vi "UI - All UI Objects Refs Memory.vi"(7 "Operation":T1, 8 "error in":errorcluster, 11 "VI Name (\"\" = Caller)":string) -> (0 "error out":errorcluster, 3 "Variant Out":variant)   [LabVIEW 2012]
uses:
  Controls/UI - All UI Objects Refs Memory - Operation.ctl
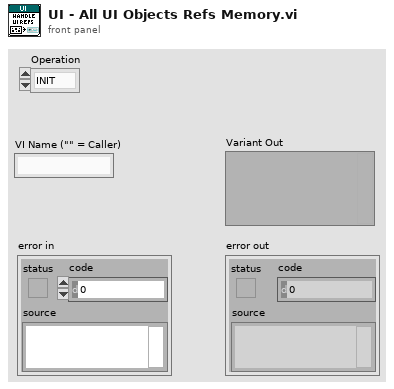
[diagram p1: front panel]
types:
  T1 = typedef "UI - All UI Objects Refs Memory - Operation.ctl" = enum16{"INIT", "GET", "ADD"}
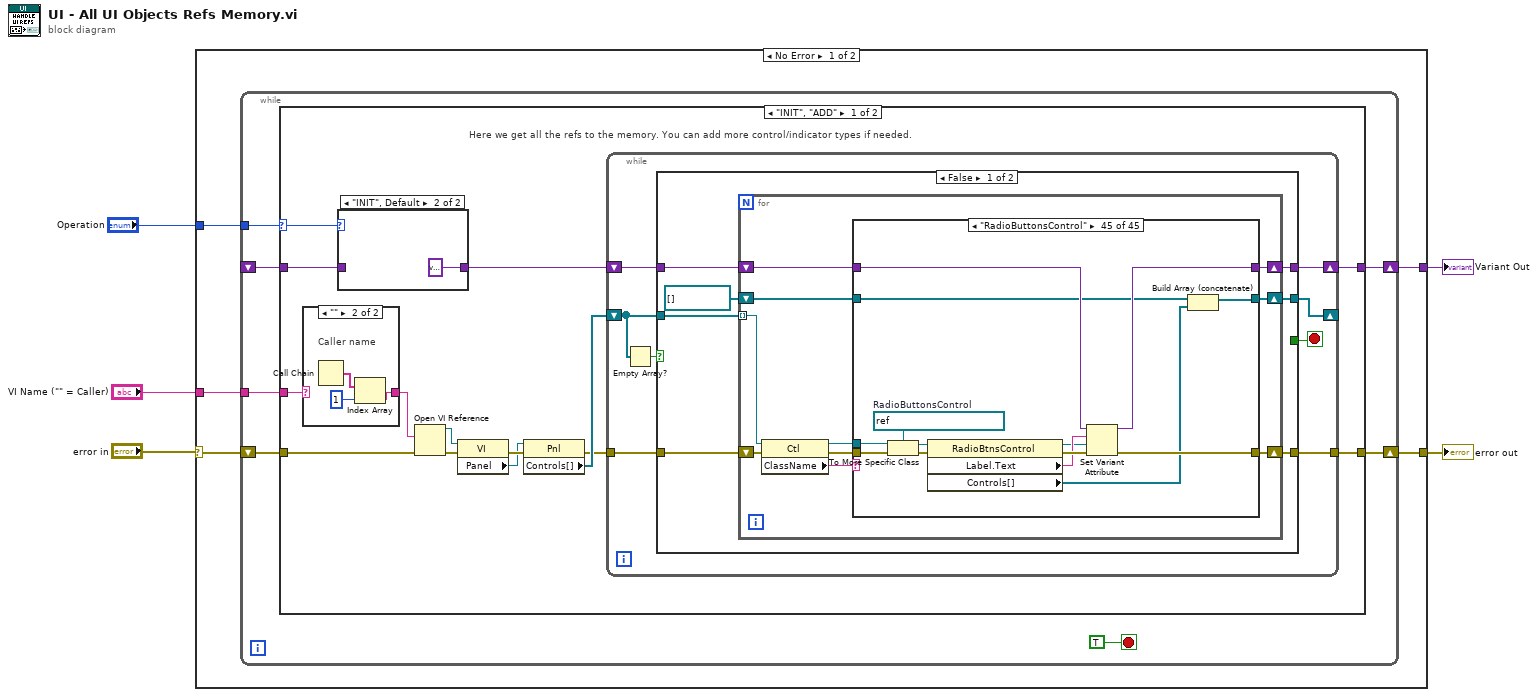
[diagram p0: block diagram]
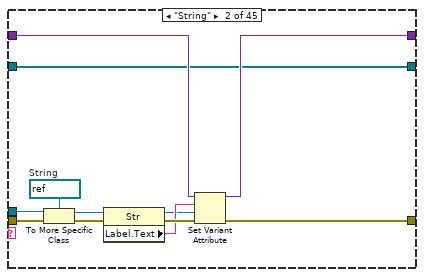
[diagram p3: hidden frame]
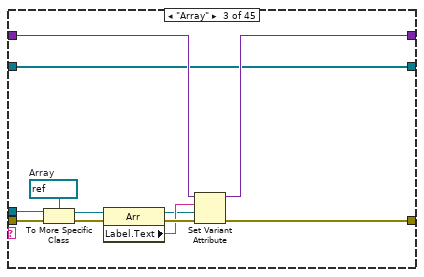
[diagram p4: hidden frame]
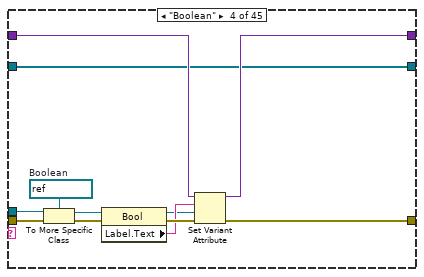
[diagram p5: hidden frame]
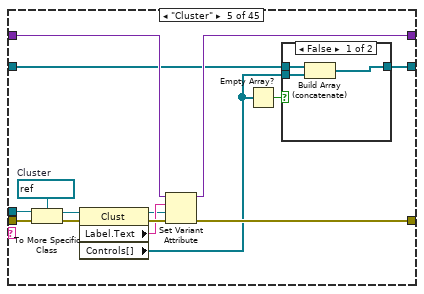
[diagram p6: hidden frame]
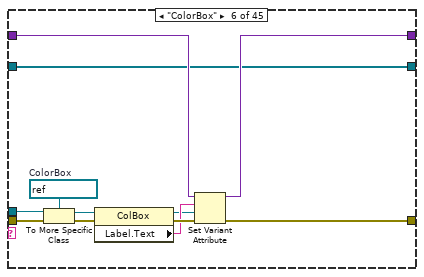
[diagram p8: hidden frame]
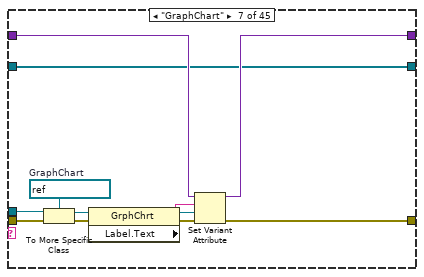
[diagram p9: hidden frame]
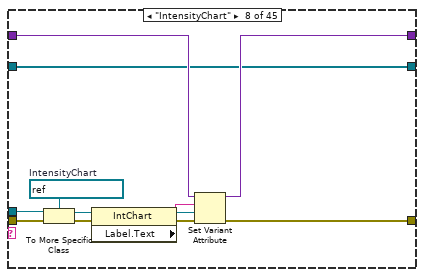
[diagram p10: hidden frame]
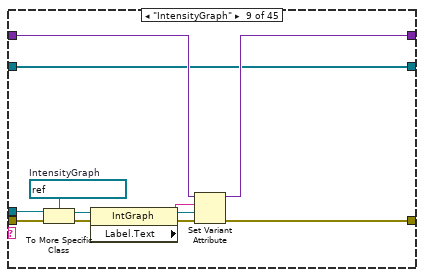
[diagram p11: hidden frame]
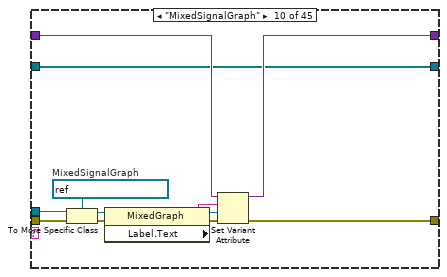
[diagram p12: hidden frame]
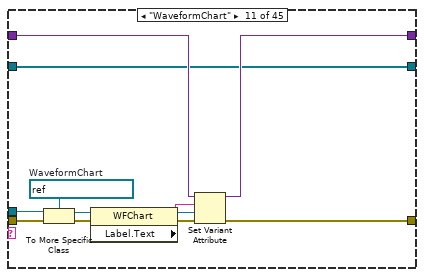
[diagram p13: hidden frame]
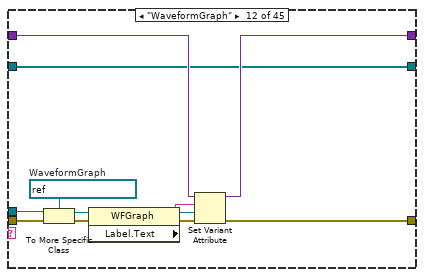
[diagram p14: hidden frame]
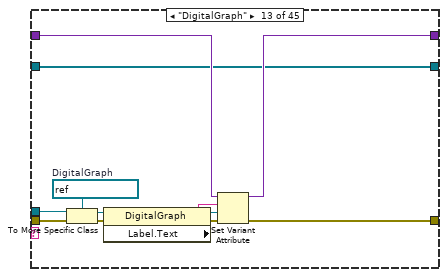
[diagram p15: hidden frame]
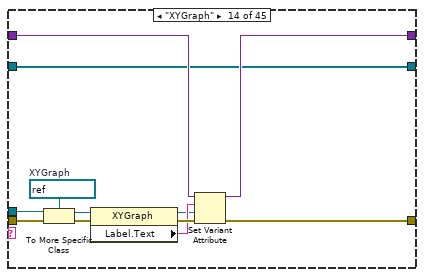
[diagram p16: hidden frame]
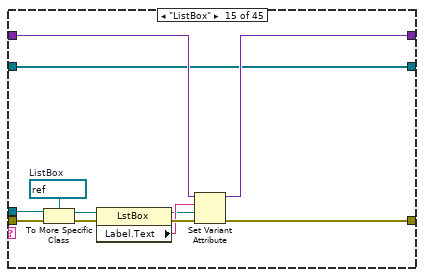
[diagram p17: hidden frame]
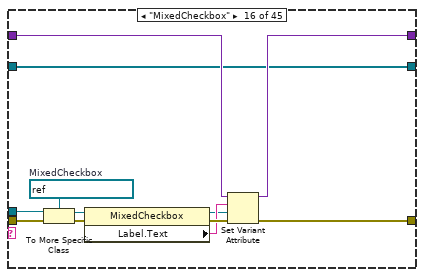
[diagram p18: hidden frame]
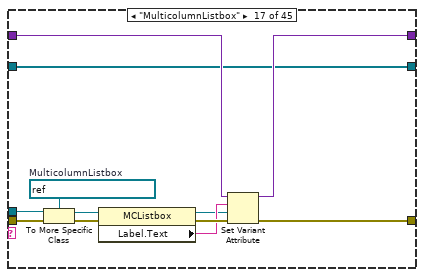
[diagram p19: hidden frame]
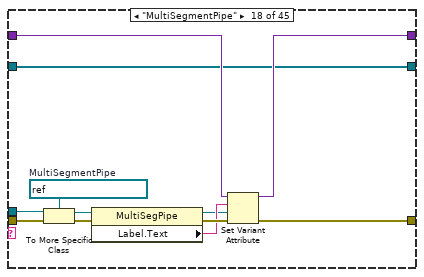
[diagram p20: hidden frame]
diagram:
  n1 = case shown="No Error" "error in" {
    selector: "error in" -> [w9 w617]
    tunnel: [w8 w617] -> w5
    tunnel: "Operation" -> [w10 _]
    tunnel: "VI Name (\"\" = Caller)" -> [w7 _]
    tunnel: [w6 _] -> w1
    frame No Error {
      n2 = while {
        tunnel: w10 -> [w16]
        shift-right: [w11] -> w8
        shift-left: w9 -> [w15]
        tunnel: w7 -> [w14]
        shift-right: [w13] -> w6
        shift-left: _ -> [w12]
        stop <- TRUE stop-if-true
        n3 = case shown="\"INIT\", \"ADD\"" w16 {
          selector: w16 -> [w20 _]
          tunnel: w15 -> [w31 w616]
          tunnel: w14 -> [w30 _]
          tunnel: [w22 w615] -> w13
          tunnel: w12 -> [w18 w615]
          tunnel: [w21 w616] -> w11
          frame "INIT", "ADD" {
            # "Here we get all the refs to the memory. You can add more control/indicator types if needed."
            n4 = case shown="\"\"" w30 {
              selector: w30 -> [w611 _]
              tunnel: [w611 w612] -> w29
              frame Default {
              }
              frame "" {
                # "Caller name"
                n5 = Call Chain() -> (call chain=w614:string[])
                n6 = Index Array(array=w614, index=1) -> (element=w612:string)
              }
            }
            n7 = case shown="\"INIT\", Default" w20 {
              tunnel: [w609 variant] -> w19
              tunnel: w18 -> [w609 _]
              frame "ADD" {
              }
              frame "INIT", Default {
              }
            }
            n8 = Open VI Reference(vi path=w29, error in (no error)=w31) -> (vi reference=w27:refnum<vi>, error out=w28:errorcluster)  [unwired: 4 in]
            n9 = property class="VI"(reference=w27, error in=w28) -> (error out=w26:errorcluster, "Panel"=w25:refnum<vi>)  [unwired: 1 out]
            n10 = property class="Pnl"(reference=w25, error in=w26) -> (error out=w23:errorcluster, "Controls[]"=w24:refnum<vi>[])  [unwired: 1 out]
            n11 = while {
              tunnel: w23 -> [w39]
              tunnel: [w37] -> w21
              shift-right: [w35] -> _
              shift-left: w24 -> [w34]
              shift-right: [w38] -> w22
              shift-left: w19 -> [w36]
              stop <- w32 stop-if-true
              n12 = Empty Array?(array=w34) -> (empty?=w33:bool)
              n13 = case shown="False" w33 {
                tunnel: w34 -> [w46 _]
                tunnel: w39 -> [w45 w608]
                tunnel: [w44 w607] -> w38
                tunnel: [w43 w608] -> w37
                tunnel: w36 -> [w42 w607]
                tunnel: [w41 _] -> w35
                tunnel: [_ TRUE] -> w32
                frame False {
                  n14 = for {
                    tunnel: w46 -> [w55] mode=indexing
                    shift-right: [w49] -> w43
                    shift-left: w45 -> [w56]
                    shift-right: [w51] -> w44
                    shift-left: w42 -> [w50]
                    shift-right: [w48] -> w41
                    shift-left: refnum<vi>[] [] ("Controls[]") -> [w47]
                    n15 = property class="Ctl"(reference=w55, error in=w56) -> (reference out=w52:refnum<vi>, error out=w54:errorcluster, "ClassName"=w53:string)
                    n16 = case shown="\"RadioButtonsControl\"" w53 {
                      tunnel: w54 -> [w58 w71 w83 w95 w110 w126 w138 w150 w162 w174 w186 w198 w210 w222 w234 w246 w258 w270 w282 w294 w306 w318 w330 w342 w354 w366 w378 w390 w405 w423 w435 w447 w459 w471 w483 w495 w507 w519 w531 w543 w555 w567 w579 w591 w605]
                      tunnel: w52 -> [_ w70 w82 w94 w109 w125 w137 w149 w161 w173 w185 w197 w209 w221 w233 w245 w257 w269 w281 w293 w305 w317 w329 w341 w353 w365 w377 w389 w404 w422 w434 w446 w458 w470 w482 w494 w506 w518 w530 w542 w554 w566 w578 w590 w604]
                      tunnel: [w59 w65 w77 w89 w104 w120 w132 w144 w156 w168 w180 w192 w204 w216 w228 w240 w252 w264 w276 w288 w300 w312 w324 w336 w348 w360 w372 w384 w399 w417 w429 w441 w453 w465 w477 w489 w501 w513 w525 w537 w549 w561 w573 w585 w599] -> w51
                      tunnel: w50 -> [w59 w64 w76 w88 w103 w119 w131 w143 w155 w167 w179 w191 w203 w215 w227 w239 w251 w263 w275 w287 w299 w311 w323 w335 w347 w359 w371 w383 w398 w416 w428 w440 w452 w464 w476 w488 w500 w512 w524 w536 w548 w560 w572 w584 w598]
                      tunnel: [w58 w61 w73 w85 w100 w116 w128 w140 w152 w164 w176 w188 w200 w212 w224 w236 w248 w260 w272 w284 w296 w308 w320 w332 w344 w356 w368 w380 w393 w413 w425 w437 w449 w461 w473 w485 w497 w509 w521 w533 w545 w557 w569 w581 w595] -> w49
                      tunnel: [w57 w60 w72 w84 w99 w115 w127 w139 w151 w163 w175 w187 w199 w211 w223 w235 w247 w259 w271 w283 w295 w307 w319 w331 w343 w355 w367 w379 w391 w412 w424 w436 w448 w460 w472 w484 w496 w508 w520 w532 w544 w556 w568 w580 w592] -> w48
                      tunnel: w47 -> [w57 w60 w72 w84 w98 w115 w127 w139 w151 w163 w175 w187 w199 w211 w223 w235 w247 w259 w271 w283 w295 w307 w319 w331 w343 w355 w367 w379 w392 w412 w424 w436 w448 w460 w472 w484 w496 w508 w520 w532 w544 w556 w568 w580 w593]
                      frame Default {
                        # "Not implemented"
                      }
                      frame "String" {
                        w67 = refnum<vi> refnum  # String
                        n17 = To More Specific Class(target class=w67, reference=w70, error in=w71) -> (specific class reference=w69:refnum<vi>, error out=w68:errorcluster)
                        n18 = property class="Str"(reference=w69, error in=w68) -> (reference out=w62:refnum<vi>, error out=w66:errorcluster, "Label.Text"=w63:string)
                        n19 = Set Variant Attribute(Variant=w64, name=w63, value=w62, error in=w66) -> (Variant out=w65:variant, error out=w61:errorcluster)  [unwired: 1 out]
                      }
                      frame "Array" {
                        w79 = refnum<vi> refnum  # Array
                        n20 = To More Specific Class(target class=w79, reference=w82, error in=w83) -> (specific class reference=w81:refnum<vi>, error out=w80:errorcluster)
                        n21 = property class="Arr"(reference=w81, error in=w80) -> (reference out=w74:refnum<vi>, error out=w78:errorcluster, "Label.Text"=w75:string)
                        n22 = Set Variant Attribute(Variant=w76, name=w75, value=w74, error in=w78) -> (Variant out=w77:variant, error out=w73:errorcluster)  [unwired: 1 out]
                      }
                      frame "Boolean" {
                        w91 = refnum<vi> refnum  # Boolean
                        n23 = To More Specific Class(target class=w91, reference=w94, error in=w95) -> (specific class reference=w93:refnum<vi>, error out=w92:errorcluster)
                        n24 = property class="Bool"(reference=w93, error in=w92) -> (reference out=w86:refnum<vi>, error out=w90:errorcluster, "Label.Text"=w87:string)
                        n25 = Set Variant Attribute(Variant=w88, name=w87, value=w86, error in=w90) -> (Variant out=w89:variant, error out=w85:errorcluster)  [unwired: 1 out]
                      }
                      frame "Cluster" {
                        w106 = refnum<vi> refnum  # Cluster
                        n26 = To More Specific Class(target class=w106, reference=w109, error in=w110) -> (specific class reference=w108:refnum<vi>, error out=w107:errorcluster)
                        n27 = property class="Clust"(reference=w108, error in=w107) -> (reference out=w101:refnum<vi>, error out=w105:errorcluster, "Label.Text"=w102:string, "Controls[]"=w97:refnum<vi>[])
                        n28 = Set Variant Attribute(Variant=w103, name=w102, value=w101, error in=w105) -> (Variant out=w104:variant, error out=w100:errorcluster)  [unwired: 1 out]
                        n29 = Empty Array?(array=w97) -> (empty?=w96:bool)
                        n30 = case shown="False" w96 {
                          tunnel: w97 -> [w113 _]
                          tunnel: [w112 w114] -> w99
                          tunnel: w98 -> [w111 w114]
                          frame False {
                            n31 = Build Array (concatenate)(w111, w113) -> (w112:refnum<vi>[])
                          }
                          frame True {
                          }
                        }
                      }
                      frame "ColorBox" {
                        w122 = refnum<vi> refnum  # ColorBox
                        n32 = To More Specific Class(target class=w122, reference=w125, error in=w126) -> (specific class reference=w124:refnum<vi>, error out=w123:errorcluster)
                        n33 = property class="ColBox"(reference=w124, error in=w123) -> (reference out=w117:refnum<vi>, error out=w121:errorcluster, "Label.Text"=w118:string)
                        n34 = Set Variant Attribute(Variant=w119, name=w118, value=w117, error in=w121) -> (Variant out=w120:variant, error out=w116:errorcluster)  [unwired: 1 out]
                      }
                      frame "GraphChart" {
                        w134 = refnum<vi> refnum  # GraphChart
                        n35 = To More Specific Class(target class=w134, reference=w137, error in=w138) -> (specific class reference=w136:refnum<vi>, error out=w135:errorcluster)
                        n36 = property class="GrphChrt"(reference=w136, error in=w135) -> (reference out=w129:refnum<vi>, error out=w133:errorcluster, "Label.Text"=w130:string)
                        n37 = Set Variant Attribute(Variant=w131, name=w130, value=w129, error in=w133) -> (Variant out=w132:variant, error out=w128:errorcluster)  [unwired: 1 out]
                      }
                      frame "IntensityChart" {
                        w146 = refnum<vi> refnum  # IntensityChart
                        n38 = To More Specific Class(target class=w146, reference=w149, error in=w150) -> (specific class reference=w148:refnum<vi>, error out=w147:errorcluster)
                        n39 = property class="IntChart"(reference=w148, error in=w147) -> (reference out=w141:refnum<vi>, error out=w145:errorcluster, "Label.Text"=w142:string)
                        n40 = Set Variant Attribute(Variant=w143, name=w142, value=w141, error in=w145) -> (Variant out=w144:variant, error out=w140:errorcluster)  [unwired: 1 out]
                      }
                      frame "IntensityGraph" {
                        w158 = refnum<vi> refnum  # IntensityGraph
                        n41 = To More Specific Class(target class=w158, reference=w161, error in=w162) -> (specific class reference=w160:refnum<vi>, error out=w159:errorcluster)
                        n42 = property class="IntGraph"(reference=w160, error in=w159) -> (reference out=w153:refnum<vi>, error out=w157:errorcluster, "Label.Text"=w154:string)
                        n43 = Set Variant Attribute(Variant=w155, name=w154, value=w153, error in=w157) -> (Variant out=w156:variant, error out=w152:errorcluster)  [unwired: 1 out]
                      }
                      frame "MixedSignalGraph" {
                        w170 = refnum<vi> refnum  # MixedSignalGraph
                        n44 = To More Specific Class(target class=w170, reference=w173, error in=w174) -> (specific class reference=w172:refnum<vi>, error out=w171:errorcluster)
                        n45 = property class="MixedGraph"(reference=w172, error in=w171) -> (reference out=w165:refnum<vi>, error out=w169:errorcluster, "Label.Text"=w166:string)
                        n46 = Set Variant Attribute(Variant=w167, name=w166, value=w165, error in=w169) -> (Variant out=w168:variant, error out=w164:errorcluster)  [unwired: 1 out]
                      }
                      frame "WaveformChart" {
                        w182 = refnum<vi> refnum  # WaveformChart
                        n47 = To More Specific Class(target class=w182, reference=w185, error in=w186) -> (specific class reference=w184:refnum<vi>, error out=w183:errorcluster)
                        n48 = property class="WFChart"(reference=w184, error in=w183) -> (reference out=w177:refnum<vi>, error out=w181:errorcluster, "Label.Text"=w178:string)
                        n49 = Set Variant Attribute(Variant=w179, name=w178, value=w177, error in=w181) -> (Variant out=w180:variant, error out=w176:errorcluster)  [unwired: 1 out]
                      }
                      frame "WaveformGraph" {
                        w194 = refnum<vi> refnum  # WaveformGraph
                        n50 = To More Specific Class(target class=w194, reference=w197, error in=w198) -> (specific class reference=w196:refnum<vi>, error out=w195:errorcluster)
                        n51 = property class="WFGraph"(reference=w196, error in=w195) -> (reference out=w189:refnum<vi>, error out=w193:errorcluster, "Label.Text"=w190:string)
                        n52 = Set Variant Attribute(Variant=w191, name=w190, value=w189, error in=w193) -> (Variant out=w192:variant, error out=w188:errorcluster)  [unwired: 1 out]
                      }
                      frame "DigitalGraph" {
                        w206 = refnum<vi> refnum  # DigitalGraph
                        n53 = To More Specific Class(target class=w206, reference=w209, error in=w210) -> (specific class reference=w208:refnum<vi>, error out=w207:errorcluster)
                        n54 = property class="DigitalGraph"(reference=w208, error in=w207) -> (reference out=w201:refnum<vi>, error out=w205:errorcluster, "Label.Text"=w202:string)
                        n55 = Set Variant Attribute(Variant=w203, name=w202, value=w201, error in=w205) -> (Variant out=w204:variant, error out=w200:errorcluster)  [unwired: 1 out]
                      }
                      frame "XYGraph" {
                        w218 = refnum<vi> refnum  # XYGraph
                        n56 = To More Specific Class(target class=w218, reference=w221, error in=w222) -> (specific class reference=w220:refnum<vi>, error out=w219:errorcluster)
                        n57 = property class="XYGraph"(reference=w220, error in=w219) -> (reference out=w213:refnum<vi>, error out=w217:errorcluster, "Label.Text"=w214:string)
                        n58 = Set Variant Attribute(Variant=w215, name=w214, value=w213, error in=w217) -> (Variant out=w216:variant, error out=w212:errorcluster)  [unwired: 1 out]
                      }
                      frame "ListBox" {
                        w230 = refnum<vi> refnum  # ListBox
                        n59 = To More Specific Class(target class=w230, reference=w233, error in=w234) -> (specific class reference=w232:refnum<vi>, error out=w231:errorcluster)
                        n60 = property class="LstBox"(reference=w232, error in=w231) -> (reference out=w225:refnum<vi>, error out=w229:errorcluster, "Label.Text"=w226:string)
                        n61 = Set Variant Attribute(Variant=w227, name=w226, value=w225, error in=w229) -> (Variant out=w228:variant, error out=w224:errorcluster)  [unwired: 1 out]
                      }
                      frame "MixedCheckbox" {
                        w242 = refnum<vi> refnum  # MixedCheckbox
                        n62 = To More Specific Class(target class=w242, reference=w245, error in=w246) -> (specific class reference=w244:refnum<vi>, error out=w243:errorcluster)
                        n63 = property class="MixedCheckbox"(reference=w244, error in=w243) -> (reference out=w237:refnum<vi>, error out=w241:errorcluster, "Label.Text"=w238:string)
                        n64 = Set Variant Attribute(Variant=w239, name=w238, value=w237, error in=w241) -> (Variant out=w240:variant, error out=w236:errorcluster)  [unwired: 1 out]
                      }
                      frame "MulticolumnListbox" {
                        w254 = refnum<vi> refnum  # MulticolumnListbox
                        n65 = To More Specific Class(target class=w254, reference=w257, error in=w258) -> (specific class reference=w256:refnum<vi>, error out=w255:errorcluster)
                        n66 = property class="MCListbox"(reference=w256, error in=w255) -> (reference out=w249:refnum<vi>, error out=w253:errorcluster, "Label.Text"=w250:string)
                        n67 = Set Variant Attribute(Variant=w251, name=w250, value=w249, error in=w253) -> (Variant out=w252:variant, error out=w248:errorcluster)  [unwired: 1 out]
                      }
                      frame "MultiSegmentPipe" {
                        w266 = refnum<vi> refnum  # MultiSegmentPipe
                        n68 = To More Specific Class(target class=w266, reference=w269, error in=w270) -> (specific class reference=w268:refnum<vi>, error out=w267:errorcluster)
                        n69 = property class="MultiSegPipe"(reference=w268, error in=w267) -> (reference out=w261:refnum<vi>, error out=w265:errorcluster, "Label.Text"=w262:string)
                        n70 = Set Variant Attribute(Variant=w263, name=w262, value=w261, error in=w265) -> (Variant out=w264:variant, error out=w260:errorcluster)  [unwired: 1 out]
                      }
                      frame "Numeric" {
                        w278 = refnum<vi> refnum  # Numeric
                        n71 = To More Specific Class(target class=w278, reference=w281, error in=w282) -> (specific class reference=w280:refnum<vi>, error out=w279:errorcluster)
                        n72 = property class="Num"(reference=w280, error in=w279) -> (reference out=w273:refnum<vi>, error out=w277:errorcluster, "Label.Text"=w274:string)
                        n73 = Set Variant Attribute(Variant=w275, name=w274, value=w273, error in=w277) -> (Variant out=w276:variant, error out=w272:errorcluster)  [unwired: 1 out]
                      }
                      frame "ColorRamp" {
                        w290 = refnum<vi> refnum  # ColorRamp
                        n74 = To More Specific Class(target class=w290, reference=w293, error in=w294) -> (specific class reference=w292:refnum<vi>, error out=w291:errorcluster)
                        n75 = property class="ColRmp"(reference=w292, error in=w291) -> (reference out=w285:refnum<vi>, error out=w289:errorcluster, "Label.Text"=w286:string)
                        n76 = Set Variant Attribute(Variant=w287, name=w286, value=w285, error in=w289) -> (Variant out=w288:variant, error out=w284:errorcluster)  [unwired: 1 out]
                      }
                      frame "Digital" {
                        w302 = refnum<vi> refnum  # Digital
                        n77 = To More Specific Class(target class=w302, reference=w305, error in=w306) -> (specific class reference=w304:refnum<vi>, error out=w303:errorcluster)
                        n78 = property class="DigNum"(reference=w304, error in=w303) -> (reference out=w297:refnum<vi>, error out=w301:errorcluster, "Label.Text"=w298:string)
                        n79 = Set Variant Attribute(Variant=w299, name=w298, value=w297, error in=w301) -> (Variant out=w300:variant, error out=w296:errorcluster)  [unwired: 1 out]
                      }
                      frame "NamedNumeric" {
                        w314 = refnum<vi> refnum  # NamedNumeric
                        n80 = To More Specific Class(target class=w314, reference=w317, error in=w318) -> (specific class reference=w316:refnum<vi>, error out=w315:errorcluster)
                        n81 = property class="NmdNum"(reference=w316, error in=w315) -> (reference out=w309:refnum<vi>, error out=w313:errorcluster, "Label.Text"=w310:string)
                        n82 = Set Variant Attribute(Variant=w311, name=w310, value=w309, error in=w313) -> (Variant out=w312:variant, error out=w308:errorcluster)  [unwired: 1 out]
                      }
                      frame "Enum" {
                        w326 = refnum<vi> refnum  # Enum
                        n83 = To More Specific Class(target class=w326, reference=w329, error in=w330) -> (specific class reference=w328:refnum<vi>, error out=w327:errorcluster)
                        n84 = property class="Enum"(reference=w328, error in=w327) -> (reference out=w321:refnum<vi>, error out=w325:errorcluster, "Label.Text"=w322:string)
                        n85 = Set Variant Attribute(Variant=w323, name=w322, value=w321, error in=w325) -> (Variant out=w324:variant, error out=w320:errorcluster)  [unwired: 1 out]
                      }
                      frame "Ring" {
                        w338 = refnum<vi> refnum  # Ring
                        n86 = To More Specific Class(target class=w338, reference=w341, error in=w342) -> (specific class reference=w340:refnum<vi>, error out=w339:errorcluster)
                        n87 = property class="Ring"(reference=w340, error in=w339) -> (reference out=w333:refnum<vi>, error out=w337:errorcluster, "Label.Text"=w334:string)
                        n88 = Set Variant Attribute(Variant=w335, name=w334, value=w333, error in=w337) -> (Variant out=w336:variant, error out=w332:errorcluster)  [unwired: 1 out]
                      }
                      frame "NumericWithScale" {
                        w350 = refnum<vi> refnum  # NumericWithScale
                        n89 = To More Specific Class(target class=w350, reference=w353, error in=w354) -> (specific class reference=w352:refnum<vi>, error out=w351:errorcluster)
                        n90 = property class="NumWthScl"(reference=w352, error in=w351) -> (reference out=w345:refnum<vi>, error out=w349:errorcluster, "Label.Text"=w346:string)
                        n91 = Set Variant Attribute(Variant=w347, name=w346, value=w345, error in=w349) -> (Variant out=w348:variant, error out=w344:errorcluster)  [unwired: 1 out]
                      }
                      frame "Knob" {
                        w362 = refnum<vi> refnum  # Knob
                        n92 = To More Specific Class(target class=w362, reference=w365, error in=w366) -> (specific class reference=w364:refnum<vi>, error out=w363:errorcluster)
                        n93 = property class="Knob"(reference=w364, error in=w363) -> (reference out=w357:refnum<vi>, error out=w361:errorcluster, "Label.Text"=w358:string)
                        n94 = Set Variant Attribute(Variant=w359, name=w358, value=w357, error in=w361) -> (Variant out=w360:variant, error out=w356:errorcluster)  [unwired: 1 out]
                      }
                      frame "Slide" {
                        w374 = refnum<vi> refnum  # Slide
                        n95 = To More Specific Class(target class=w374, reference=w377, error in=w378) -> (specific class reference=w376:refnum<vi>, error out=w375:errorcluster)
                        n96 = property class="Slide"(reference=w376, error in=w375) -> (reference out=w369:refnum<vi>, error out=w373:errorcluster, "Label.Text"=w370:string)
                        n97 = Set Variant Attribute(Variant=w371, name=w370, value=w369, error in=w373) -> (Variant out=w372:variant, error out=w368:errorcluster)  [unwired: 1 out]
                      }
                      frame "PageSelector" {
                        w386 = refnum<vi> refnum  # PageSelector
                        n98 = To More Specific Class(target class=w386, reference=w389, error in=w390) -> (specific class reference=w388:refnum<vi>, error out=w387:errorcluster)
                        n99 = property class="PageSel"(reference=w388, error in=w387) -> (reference out=w381:refnum<vi>, error out=w385:errorcluster, "Label.Text"=w382:string)
                        n100 = Set Variant Attribute(Variant=w383, name=w382, value=w381, error in=w385) -> (Variant out=w384:variant, error out=w380:errorcluster)  [unwired: 1 out]
                      }
                      frame "TabControl" {
                        w401 = refnum<vi> refnum  # TabControl
                        n101 = To More Specific Class(target class=w401, reference=w404, error in=w405) -> (specific class reference=w403:refnum<vi>, error out=w402:errorcluster)
                        n102 = property class="TabCtl"(reference=w403, error in=w402) -> (reference out=w396:refnum<vi>, error out=w400:errorcluster, "Label.Text"=w397:string, "Pages"=w394:refnum<vi>[])
                        n103 = Set Variant Attribute(Variant=w398, name=w397, value=w396, error in=w400) -> (Variant out=w399:variant, error out=w395:errorcluster)  [unwired: 1 out]
                        n104 = for {
                          tunnel: w394 -> [w410] mode=indexing
                          shift-right: [w409] -> w393
                          shift-left: w395 -> [w411]
                          shift-right: [w406] -> w391
                          shift-left: w392 -> [w408]
                          n105 = property class="Page"(reference=w410, error in=w411) -> (error out=w409:errorcluster, "ControlsOnPage"=w407:refnum<vi>[])  [unwired: 1 out]
                          n106 = Build Array (concatenate)(w408, w407) -> (w406:refnum<vi>[])
                        }
                      }
                      frame "Path" {
                        w419 = refnum<vi> refnum  # Path
                        n107 = To More Specific Class(target class=w419, reference=w422, error in=w423) -> (specific class reference=w421:refnum<vi>, error out=w420:errorcluster)
                        n108 = property class="Path"(reference=w421, error in=w420) -> (reference out=w414:refnum<vi>, error out=w418:errorcluster, "Label.Text"=w415:string)
                        n109 = Set Variant Attribute(Variant=w416, name=w415, value=w414, error in=w418) -> (Variant out=w417:variant, error out=w413:errorcluster)  [unwired: 1 out]
                      }
                      frame "Picture" {
                        w431 = refnum<vi> refnum  # Picture
                        n110 = To More Specific Class(target class=w431, reference=w434, error in=w435) -> (specific class reference=w433:refnum<vi>, error out=w432:errorcluster)
                        n111 = property class="Pict"(reference=w433, error in=w432) -> (reference out=w426:refnum<vi>, error out=w430:errorcluster, "Label.Text"=w427:string)
                        n112 = Set Variant Attribute(Variant=w428, name=w427, value=w426, error in=w430) -> (Variant out=w429:variant, error out=w425:errorcluster)  [unwired: 1 out]
                      }
                      frame "Pixmap" {
                        w443 = refnum<vi> refnum  # Pixmap
                        n113 = To More Specific Class(target class=w443, reference=w446, error in=w447) -> (specific class reference=w445:refnum<vi>, error out=w444:errorcluster)
                        n114 = property class="Pixmap"(reference=w445, error in=w444) -> (reference out=w438:refnum<vi>, error out=w442:errorcluster, "Label.Text"=w439:string)
                        n115 = Set Variant Attribute(Variant=w440, name=w439, value=w438, error in=w442) -> (Variant out=w441:variant, error out=w437:errorcluster)  [unwired: 1 out]
                      }
                      frame "RefNum" {
                        w455 = refnum<vi> refnum  # RefNum
                        n116 = To More Specific Class(target class=w455, reference=w458, error in=w459) -> (specific class reference=w457:refnum<vi>, error out=w456:errorcluster)
                        n117 = property class="Ref"(reference=w457, error in=w456) -> (reference out=w450:refnum<vi>, error out=w454:errorcluster, "Label.Text"=w451:string)
                        n118 = Set Variant Attribute(Variant=w452, name=w451, value=w450, error in=w454) -> (Variant out=w453:variant, error out=w449:errorcluster)  [unwired: 1 out]
                      }
                      frame "LVObjectRefNum" {
                        w467 = refnum<vi> refnum  # LVObjectRefNum
                        n119 = To More Specific Class(target class=w467, reference=w470, error in=w471) -> (specific class reference=w469:refnum<vi>, error out=w468:errorcluster)
                        n120 = property class="LVObjRef"(reference=w469, error in=w468) -> (reference out=w462:refnum<vi>, error out=w466:errorcluster, "Label.Text"=w463:string)
                        n121 = Set Variant Attribute(Variant=w464, name=w463, value=w462, error in=w466) -> (Variant out=w465:variant, error out=w461:errorcluster)  [unwired: 1 out]
                      }
                      frame "VIRefNum" {
                        w479 = refnum<vi> refnum  # VIRefNum
                        n122 = To More Specific Class(target class=w479, reference=w482, error in=w483) -> (specific class reference=w481:refnum<vi>, error out=w480:errorcluster)
                        n123 = property class="VIRef"(reference=w481, error in=w480) -> (reference out=w474:refnum<vi>, error out=w478:errorcluster, "Label.Text"=w475:string)
                        n124 = Set Variant Attribute(Variant=w476, name=w475, value=w474, error in=w478) -> (Variant out=w477:variant, error out=w473:errorcluster)  [unwired: 1 out]
                      }
                      frame "TypedRefNum" {
                        w491 = refnum<vi> refnum  # TypedRefNum
                        n125 = To More Specific Class(target class=w491, reference=w494, error in=w495) -> (specific class reference=w493:refnum<vi>, error out=w492:errorcluster)
                        n126 = property class="TypRef"(reference=w493, error in=w492) -> (reference out=w486:refnum<vi>, error out=w490:errorcluster, "Label.Text"=w487:string)
                        n127 = Set Variant Attribute(Variant=w488, name=w487, value=w486, error in=w490) -> (Variant out=w489:variant, error out=w485:errorcluster)  [unwired: 1 out]
                      }
                      frame "DataValRefNum" {
                        w503 = refnum<vi> refnum  # DataValRefNum
                        n128 = To More Specific Class(target class=w503, reference=w506, error in=w507) -> (specific class reference=w505:refnum<vi>, error out=w504:errorcluster)
                        n129 = property class="DataValRefNum"(reference=w505, error in=w504) -> (reference out=w498:refnum<vi>, error out=w502:errorcluster, "Label.Text"=w499:string)
                        n130 = Set Variant Attribute(Variant=w500, name=w499, value=w498, error in=w502) -> (Variant out=w501:variant, error out=w497:errorcluster)  [unwired: 1 out]
                      }
                      frame "SceneGraphDisplay" {
                        w515 = refnum<vi> refnum  # SceneGraphDisplay
                        n131 = To More Specific Class(target class=w515, reference=w518, error in=w519) -> (specific class reference=w517:refnum<vi>, error out=w516:errorcluster)
                        n132 = property class="SceneGraphDisp"(reference=w517, error in=w516) -> (reference out=w510:refnum<vi>, error out=w514:errorcluster, "Label.Text"=w511:string)
                        n133 = Set Variant Attribute(Variant=w512, name=w511, value=w510, error in=w514) -> (Variant out=w513:variant, error out=w509:errorcluster)  [unwired: 1 out]
                      }
                      frame "Scrollbar" {
                        w527 = refnum<vi> refnum  # Scrollbar
                        n134 = To More Specific Class(target class=w527, reference=w530, error in=w531) -> (specific class reference=w529:refnum<vi>, error out=w528:errorcluster)
                        n135 = property class="Scroll"(reference=w529, error in=w528) -> (reference out=w522:refnum<vi>, error out=w526:errorcluster, "Label.Text"=w523:string)
                        n136 = Set Variant Attribute(Variant=w524, name=w523, value=w522, error in=w526) -> (Variant out=w525:variant, error out=w521:errorcluster)  [unwired: 1 out]
                      }
                      frame "ComboBox" {
                        w539 = refnum<vi> refnum  # ComboBox
                        n137 = To More Specific Class(target class=w539, reference=w542, error in=w543) -> (specific class reference=w541:refnum<vi>, error out=w540:errorcluster)
                        n138 = property class="CmbBox"(reference=w541, error in=w540) -> (reference out=w534:refnum<vi>, error out=w538:errorcluster, "Label.Text"=w535:string)
                        n139 = Set Variant Attribute(Variant=w536, name=w535, value=w534, error in=w538) -> (Variant out=w537:variant, error out=w533:errorcluster)  [unwired: 1 out]
                      }
                      frame "SubPanel" {
                        w551 = refnum<vi> refnum  # SubPanel
                        n140 = To More Specific Class(target class=w551, reference=w554, error in=w555) -> (specific class reference=w553:refnum<vi>, error out=w552:errorcluster)
                        n141 = property class="SubPnl" props=["Label", "Text", "DiagramInserted"](reference=w553, error in=w552) -> (reference out=w546:refnum<vi>, error out=w550:errorcluster, "Label.Text"=w547:string)  [unwired: 1 out]
                        n142 = Set Variant Attribute(Variant=w548, name=w547, value=w546, error in=w550) -> (Variant out=w549:variant, error out=w545:errorcluster)  [unwired: 1 out]
                      }
                      frame "Table" {
                        w563 = refnum<vi> refnum  # Table
                        n143 = To More Specific Class(target class=w563, reference=w566, error in=w567) -> (specific class reference=w565:refnum<vi>, error out=w564:errorcluster)
                        n144 = property class="Tbl"(reference=w565, error in=w564) -> (reference out=w558:refnum<vi>, error out=w562:errorcluster, "Label.Text"=w559:string)
                        n145 = Set Variant Attribute(Variant=w560, name=w559, value=w558, error in=w562) -> (Variant out=w561:variant, error out=w557:errorcluster)  [unwired: 1 out]
                      }
                      frame "TreeControl" {
                        w575 = refnum<vi> refnum  # TreeControl
                        n146 = To More Specific Class(target class=w575, reference=w578, error in=w579) -> (specific class reference=w577:refnum<vi>, error out=w576:errorcluster)
                        n147 = property class="Tree"(reference=w577, error in=w576) -> (reference out=w570:refnum<vi>, error out=w574:errorcluster, "Label.Text"=w571:string)
                        n148 = Set Variant Attribute(Variant=w572, name=w571, value=w570, error in=w574) -> (Variant out=w573:variant, error out=w569:errorcluster)  [unwired: 1 out]
                      }
                      frame "WaveformData" {
                        w587 = refnum<vi> refnum  # WaveformData
                        n149 = To More Specific Class(target class=w587, reference=w590, error in=w591) -> (specific class reference=w589:refnum<vi>, error out=w588:errorcluster)
                        n150 = property class="WFD"(reference=w589, error in=w588) -> (reference out=w582:refnum<vi>, error out=w586:errorcluster, "Label.Text"=w583:string)
                        n151 = Set Variant Attribute(Variant=w584, name=w583, value=w582, error in=w586) -> (Variant out=w585:variant, error out=w581:errorcluster)  [unwired: 1 out]
                      }
                      frame "RadioButtonsControl" {
                        w601 = refnum<vi> refnum  # RadioButtonsControl
                        n152 = To More Specific Class(target class=w601, reference=w604, error in=w605) -> (specific class reference=w603:refnum<vi>, error out=w602:errorcluster)
                        n153 = property class="RadioBtnsControl"(reference=w603, error in=w602) -> (reference out=w596:refnum<vi>, error out=w600:errorcluster, "Label.Text"=w597:string, "Controls[]"=w594:refnum<vi>[])
                        n154 = Set Variant Attribute(Variant=w598, name=w597, value=w596, error in=w600) -> (Variant out=w599:variant, error out=w595:errorcluster)  [unwired: 1 out]
                        n155 = Build Array (concatenate)(w593, w594) -> (w592:refnum<vi>[])
                      }
                    }
                  }
                }
                frame True {
                }
              }
            }
          }
          frame "GET" {
            # "Here we just read out the shift register..."
          }
        }
      }
    }
    frame Error {
    }
  }
  "error out" <- w5
  "Variant Out" <- w1
